vi "Set Frequency.vi"(8 "error in (no error)":errorcluster, 9 "Synchronous":bool, 10 "Frequency":dbl format="%#_6pHz", 11 "Lock-in Driver in":refnum<class "Lock-in Driver.lvclass">) -> (0 "error out":errorcluster, 2 "Actual frequency":dbl format="%#_6pHz", 3 "Lock-in Driver out":refnum<class "Lock-in Driver.lvclass">)   [LabVIEW 2016, in "Lock-in Driver.lvclass"]
uses:
  Lock-in Driver.lvclass
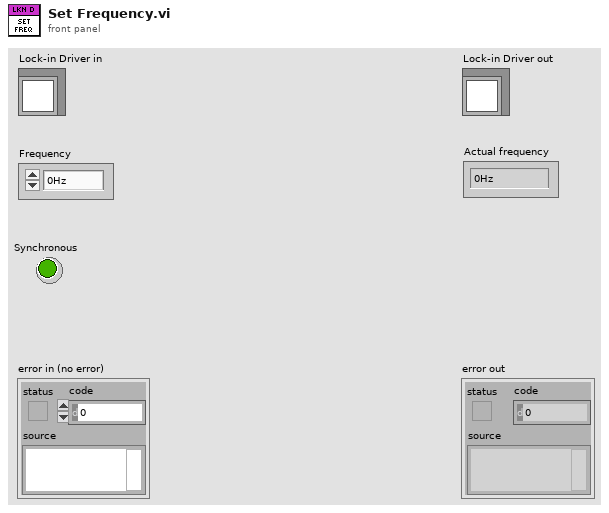
[diagram p1: front panel]
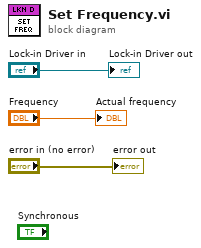
[diagram p0: block diagram]
diagram:
  "error out" <- "error in (no error)"
  "Lock-in Driver out" <- "Lock-in Driver in"
  "Actual frequency" <- "Frequency"
